vi "FindClosestPoint.vi"(8 "Y":dbl, 9 "X":dbl, 11 "Points":cluster{"X":dbl, "Y":dbl}[](graph)) -> (2 "ShortestDistanceIndex":i32, 3 "ShortestDistance":dbl)   [LabVIEW 2019]
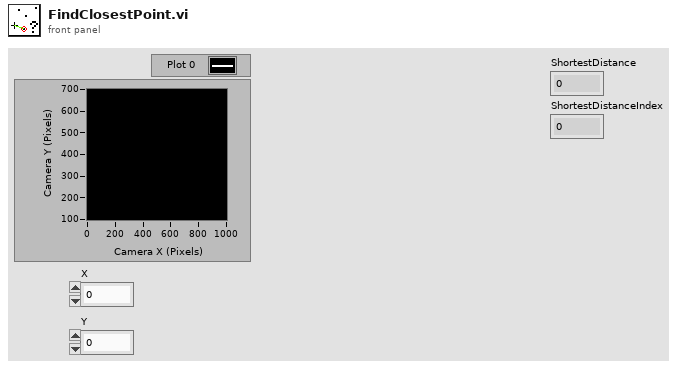
[diagram p1: front panel]
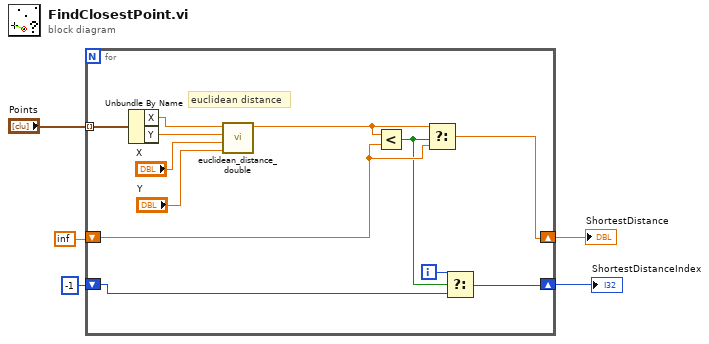
[diagram p0: block diagram]
diagram:
  n1 = for {
    tunnel: "Points" -> [w17] mode=indexing
    shift-right: [w15] -> w2
    shift-left: inf -> [w16]
    shift-right: [w14] -> w1
    shift-left: -1 -> [w11]
    i -> [w12]
    # "euclidean distance"
    n2 = Unbundle By Name(w17) -> ("X"=w10:dbl, "Y"=w9:dbl)
    n3 = call "euclidean_distance_double.vi"("Point 2 Y"="Y", "Point 2 X"="X", "Point 1 Y"=w9, "Point 1 X"=w10) -> ("Distance"=w6:dbl)  [unwired: 7 in]
    n4 = Less?(x=w6, y=w16) -> (x < y?=w13:bool)
    n5 = Select(t=w6, s=w13, f=w16) -> (s? t:f=w15:dbl)
    n6 = Select(t=w12, s=w13, f=w11) -> (s? t:f=w14:i32)
  }
  "ShortestDistance" <- w2
  "ShortestDistanceIndex" <- w1
